vi "Tablo Boya.vi"() -> ()   [LabVIEW 2014]
panel:
  out "Table Control":string[][](table)
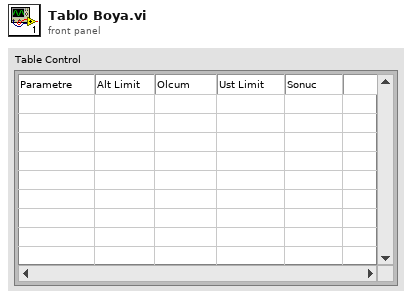
[diagram p1: front panel]
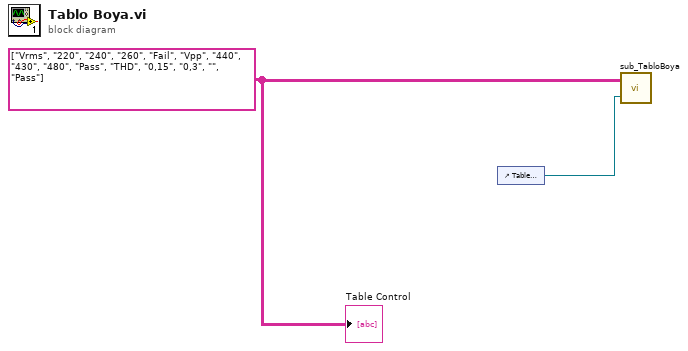
[diagram p0: block diagram]
diagram:
  w2 = string[][] [["Vrms", "220", "240", "260", "Fail"], ["Vpp", "440", "430", "480", "Pass"], ["THD", "0,15", "0,3", "", "Pass"]] ("Table Control")
  n1 = control-ref of="Table Control"() -> (w1:refnum<vi>)
  n2 = call "sub_TabloBoya.vi"("Table in"=w1, "Table Control"=w2) -> ()  [unwired: 1 in]
  "Table Control" <- w2
